vi "SIM_CurrentOutput.vi"(9 "array":dbl[][](array[numeric]), 11 "zin (m)":dbl) -> (3 "Current Out (pA)":dbl, 4 "Zread":dbl)   [LabVIEW 2017]
uses:
  <vilib>/ptbypt/NI_PtbyPt.lvlib
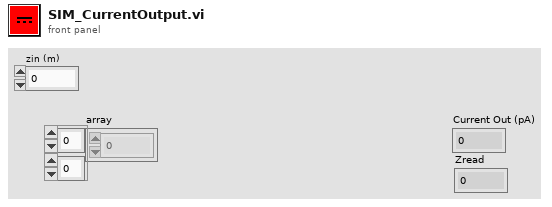
[diagram p1: front panel]
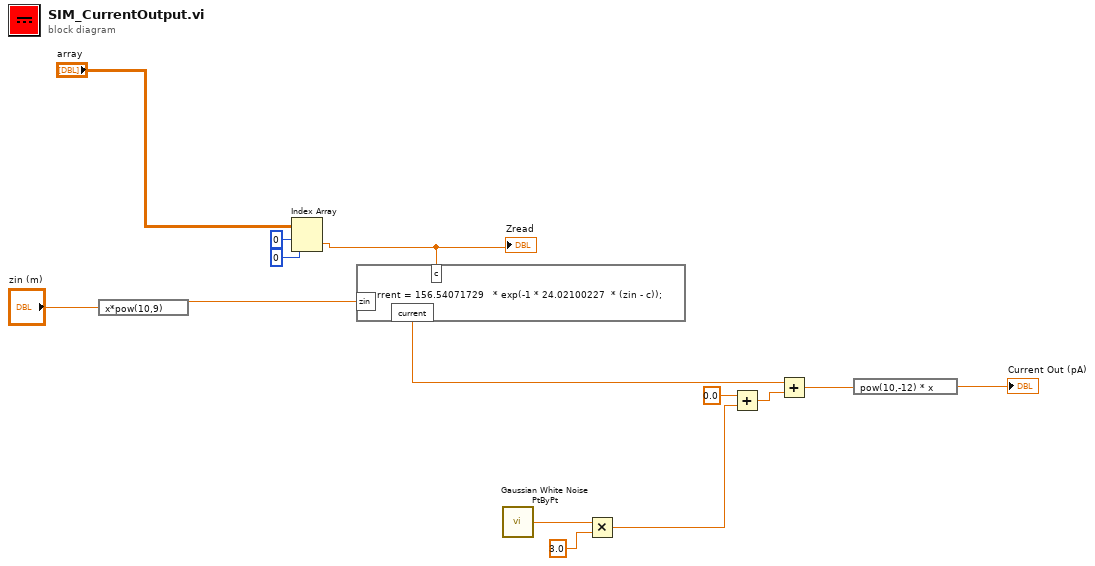
[diagram p0: block diagram]
diagram:
  n1 = expression code="x*pow(10,9)"("zin (m)") -> (w3:dbl)
  n2 = Index Array(array="array", index (row)=0, index (col)=0 ("disabled index (col)")) -> (element=w5:dbl)
  "Zread" <- w5
  n3 = formula code="current = 156.54071729   * exp(-1 * 24.02100227  * (zin - c));"("zin"=w3, "c"=w5) -> ("current"=w9:dbl)
  n4 = call <vilib>:"Gaussian White Noise PtByPt.vi"() -> ("Gaussian white noise"=w14:dbl)  [unwired: 3 in]
  n5 = Multiply(x=w14, y=3.0) -> (x*y=w11:dbl)
  n6 = Add(x=0.0, y=w11) -> (x+y=w12:dbl)
  n7 = Add(x=w9, y=w12) -> (x+y=w7:dbl)
  n8 = expression code="pow(10,-12) * x"(w7) -> (→"Current Out (pA)":dbl)
